vi "HydroHeader.vi"(0 "Comment":string, 1 "Scope":bool, 2 "File Name In":string, 3 "Votage scaling":T1={"Digitizer (dB)"=26.0, "Gain (dB)"=0.0, "Atten (dB)"=0.0}) -> (5 "Header String Out":string)   [LabVIEW 2022 SP3]
uses:
  ViewData/-ReadEye/Header.ctl
  ScanningControl/Digitizers/GaGe/-GageUtils/GageGlobals.vi
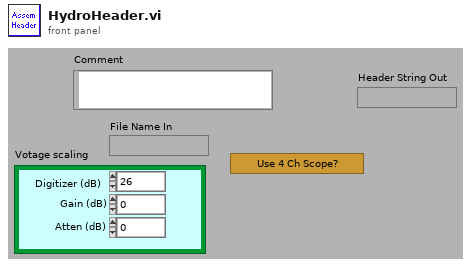
[diagram p1: front panel]
types:
  T1 = cluster{"Digitizer (dB)":sgl, "Gain (dB)":sgl, "Atten (dB)":sgl}
  T2 = typedef "Header.ctl" = cluster{"header info":cluster{"Header":string, "Head length":i16}, "A/D info":cluster{"# rf points per line":u16, "# lines per scan":u16, "sample rate MHz":u16, "# A/D bits":i16, "# bytes per A/D":u16, "TGC Flag":u16, "A/D Type":string}, "Tranducer Info":cluster{"bandwidth":sgl, "center freq":sgl, "start freq":sgl, "ID":i32}, "Scan Info":cluster{"delay":sgl, "pivot distance":sgl, "sector scan angle":sgl, "operator":string, "Scan Mode":string, "location":string}, "Time/Date Info":cluster{"date":string, "time":string}, "RF Info":cluster{"RF file name":string, "RF file att":string, "RF cal file name":string, "RF cal file att":string}, "Patient Info":cluster{"ID":string, "extended ID":string, "age":u16, "sex":string, "previously\nscanned":string, "PSA":sgl, "LOS":u8, "Ethnicty 2":u8, "Race":u8}, "Tissue Type":cluster{"organ":i16, "disease type":i16, "disease location":i16, "IQ_pts":u16, "RcvBuffer":u8, "RcvFrame":u16, "IQBuff":u8, "IQFrame":u16, "IQPage":u8}, "Votage scaling":cluster{"Digitizer (dB)":sgl, "Gain (dB)":sgl, "Atten (dB)":sgl}, "Comment":string, "Misc Info":cluster{"avg num":u16, "c speed":i16, "Div By or SF zones":i16, "XMIT CHS":u8, "RCV CHS":u8, "Xmit angle":sgl}, "Therapy Parameters":cluster{"Theraputic Freq (MHz)":sgl, "Time on (s)":sgl, "Therapy amplitude (mV)":sgl, "Lines Before":u16, "Lines After":u16}, "Scan Settings":cluster{"Energy (uJ or V)":u8, "Damp (Ohm) or Fc":u8, "HP Filt (KHz)":u8, "LP Filt (MHz)":u8, "Gain (db)":u8, "prf (kHz)":sgl, "Distance between\nscan lines (um)":u16, "Distance between\nscan planes (um)":u16, "Scan line gap (um)":sgl, "Scan plane gap (um)":sgl}, "Compression Parameters":cluster{"F1 (MHz)":sgl, "F2 (MHz)":sgl, "% taper":sgl, "duration":sgl}, "Patient Info Xtra":cluster{"First Name":string, "Last Name":string, "Notes":string}, "ROI Box":u16[]}
  T3 = cluster{"organ":i16, "disease type":i16, "disease location":i16}
  T4 = cluster{"bandwidth":sgl, "center freq":sgl, "start freq":sgl, "ID":i32}
  T5 = cluster{"# rf points per line":u16, "# lines per scan":u16, "sample rate MHz":u16, "# A/D bits":i16, "# bytes per A/D":u16, "TGC Flag":u16, "A/D Type":string}
  T6 = cluster{"Energy (microJ)":i32, "Energy (microJ)":i32, "Energy (microJ)":i32, "Energy (microJ)":i32, "Energy (microJ)":i32, "number":sgl, "number":i16, "number":i16}
  T7 = cluster{"F1 (MHz)":sgl, "F2 (MHz)":sgl, "Tukey taper":sgl, "duration":sgl}
  T8 = cluster{"delay":sgl, "pivot distance":sgl, "sector scan angle":sgl, "operator":string, "Scan Mode":string, "location":string}
  T9 = cluster{"ID":string, "extended ID":string, "age":u16, "sex":string, "previously\nscanned":string, "PSA":sgl, "LOS":u8, "Ethnicty 2":u8, "Race":u8}
  T10 = cluster{"RF file name":string, "RF file att":string, "RF cal file name":string, "RF cal file att":string}
  T11 = cluster{"avg num":i16, "c speed":i16, "Div By or SF zones":i16, "XMIT CHS":u8, "RCV CHS":u8}
  T12 = cluster{"Theraputic Freq (MHz)":sgl, "Time on (s)":sgl, "Therapy amplitude (mV)":sgl, "Lines Before":u16, "Lines After":u16}
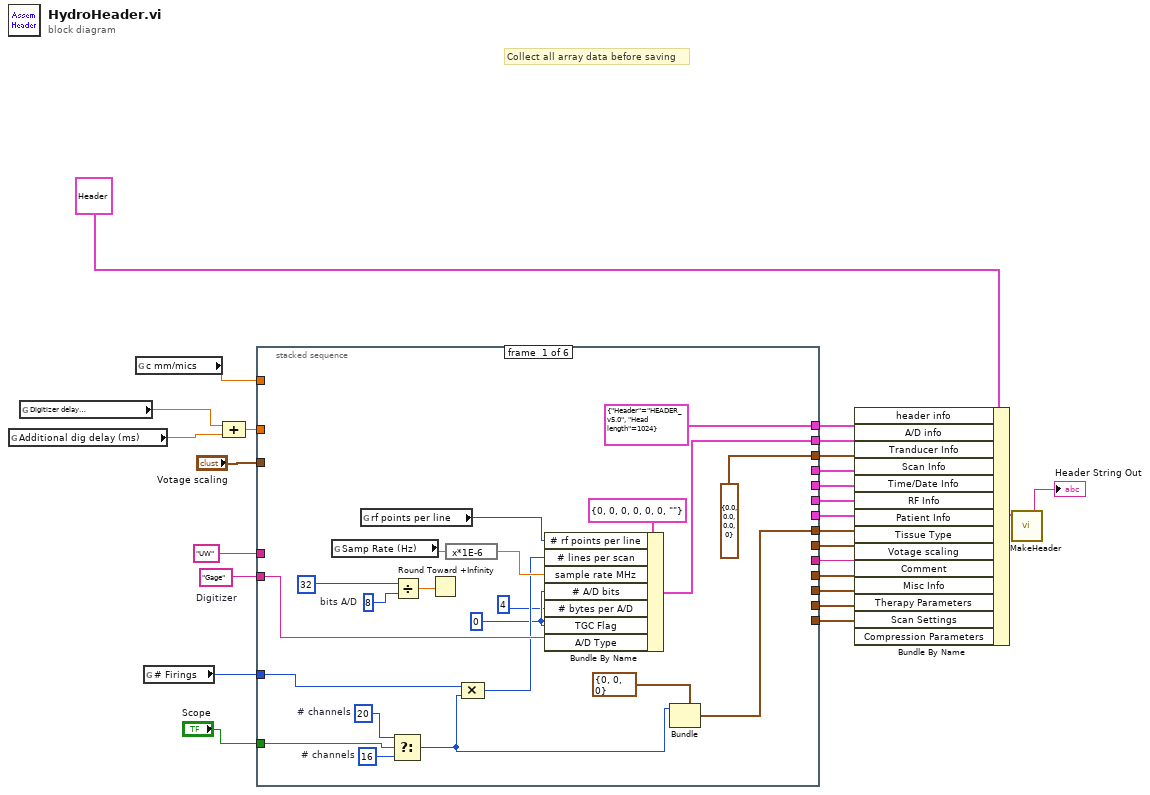
[diagram p0: block diagram]
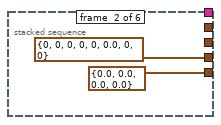
[diagram p2: hidden frame]
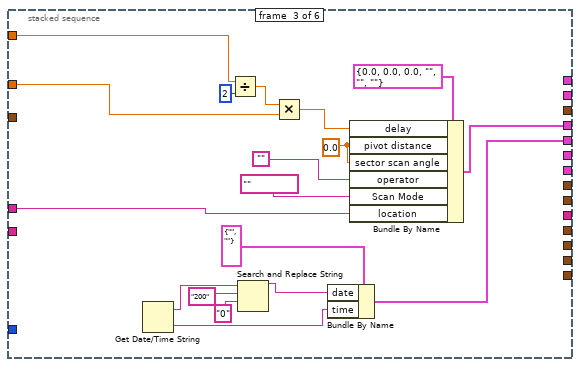
[diagram p3: hidden frame]
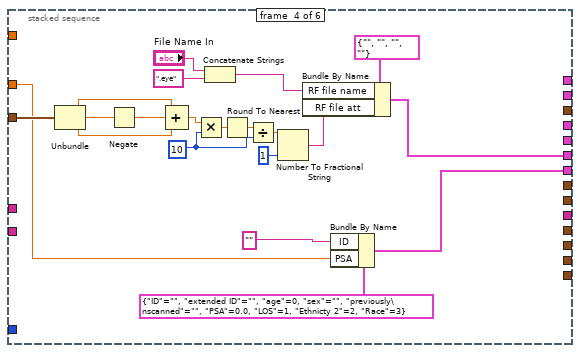
[diagram p4: hidden frame]
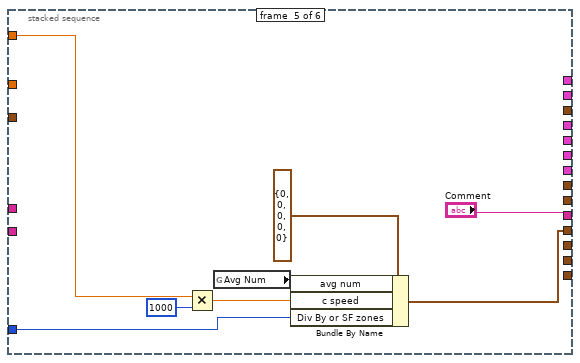
[diagram p5: hidden frame]
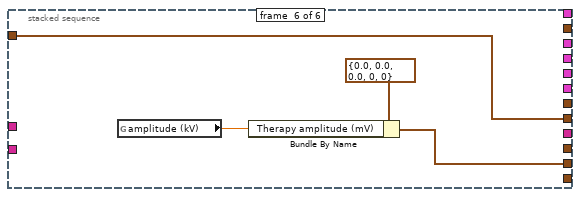
[diagram p6: hidden frame]
diagram:
  w21 = "Gage"  # Digitizer
  # "Collect all array data before saving"
  n1 = global read "GageGlobals.vi" "Additional dig delay (ms)"() -> (w4:dbl)
  n2 = global read "GageGlobals.vi" "Digitizer delay\n (ms)"() -> (w3:dbl)
  n3 = global read "GageGlobals.vi" "c mm/mics"() -> (w2:sgl)
  n4 = global read "GageGlobals.vi" "# Firings"() -> (w5:u16)
  n5 = Compound Arithmetic op=ADD(w3, w4) -> (w15:dbl)
  n6 = stacked-sequence {
    tunnel: [cluster{"Header":string, "Head length":i16} {"Header"="HEADER_v5.0", "Head length"=1024} ("header info") _ _ _ _ _] -> w26
    tunnel: [w43 _ _ _ _ _] -> w24
    tunnel: "UW" -> [_ _ w59 _ _ _]
    tunnel: [_ _ w61 _ _ _] -> w22
    tunnel: w21 -> [w42 _ _ _ _ _]
    tunnel: [T4 {"bandwidth"=0.0, "center freq"=0.0, "start freq"=0.0, "ID"=0} ("Tranducer Info") _ _ _ _ _] -> w20
    tunnel: w2 -> [_ _ w58 _ w93 _]
    tunnel: [_ _ w53 _ _ _] -> w19
    tunnel: "Votage scaling" -> [_ _ _ w70 _ w98]
    tunnel: [_ _ _ w74 _ _] -> w16
    tunnel: w15 -> [_ _ w51 w69 _ _]
    tunnel: [_ _ _ w72 _ _] -> w14
    tunnel: [_ _ _ _ _ w98] -> w13
    tunnel: [w29 _ _ _ _ _] -> w12
    tunnel: [_ _ _ _ "Comment" _] -> w11
    tunnel: [_ _ _ _ w91 _] -> w10
    tunnel: [_ _ _ _ _ w99] -> w9
    tunnel: [_ T6 {"Energy (microJ)"=0, "Energy (microJ)"=0, "Energy (microJ)"=0, "Energy (microJ)"=0, "Energy (microJ)"=0, "number"=0.0, "number"=0, "number"=0} ("output cluster") _ _ _ _] -> w8
    tunnel: [_ T7 {"F1 (MHz)"=0.0, "F2 (MHz)"=0.0, "Tukey taper"=0.0, "duration"=0.0} ("Compression Parameters") _ _ _ _] -> w7
    tunnel: w5 -> [w38 _ _ _ w90 _]
    tunnel: "Scope" -> [w32 _ _ _ _ _]
    frame #0 {
      w33 = 20  # # channels
      w34 = 16  # # channels
      w28 = u16 0 ("TGC Flag")
      w44 = 8  # bits A/D
      n7 = global read "GageGlobals.vi" "Samp Rate (Hz)"() -> (w35:dbl)
      n8 = global read "GageGlobals.vi" "rf points per line"() -> (w36:i32)
      n9 = Select(t=w33, s=w32, f=w34) -> (s? t:f=w30:i32)
      n10 = Divide(x=32, y=w44) -> (x/y=w45:dbl)
      n11 = Round Toward +Infinity(x=w45) -> ()  [unwired: 1 out]
      n12 = expression code="x*1E-6"(w35) -> (w40:dbl)
      n13 = Compound Arithmetic op=MULTIPLY(w38, w30) -> (w37:i32)
      n14 = Bundle By Name(cluster=T5 {"# rf points per line"=0, "# lines per scan"=0, "sample rate MHz"=0, "# A/D bits"=0, "# bytes per A/D"=0, "TGC Flag"=0, "A/D Type"=""} ("A/D info"), "# rf points per line"=w36, "# lines per scan"=w37, "sample rate MHz"=w40, "# A/D bits"=w28, "# bytes per A/D"=u16 4 ("TGC Flag"), "TGC Flag"=w28, "A/D Type"=w42) -> (w43:T5)
      n15 = Bundle(cluster=T3 {"organ"=0, "disease type"=0, "disease location"=0} ("Tissue Type"), "organ"=w30) -> (w29:T3)  [unwired: 2 out]
    }
    frame #1 {
    }
    frame #2 {
      w52 = sgl 0.0 ("sector scan angle")
      n16 = Get Date/Time String() -> (date string=w65:string, time string=w63:string)  [unwired: 3 out]
      n17 = Divide(x=w58, y=2) -> (x/y=w57:sgl)
      n18 = Search and Replace String(input string=w65, search string="200", replace string="0") -> (result string=w62:string)  [unwired: 1 in, 7 out]
      n19 = Multiply(x=w57, y=w51) -> (x*y=w56:dbl)
      n20 = Bundle By Name(cluster=cluster{"date":string, "time":string} {"date"="", "time"=""} ("Time/Date Info"), "date"=w62, "time"=w63) -> (w61:cluster{"date":string, "time":string})
      n21 = Bundle By Name(cluster=T8 {"delay"=0.0, "pivot distance"=0.0, "sector scan angle"=0.0, "operator"="", "Scan Mode"="", "location"=""} ("Scan Info"), "delay"=w56, "pivot distance"=w52, "sector scan angle"=w52, "operator"="", "Scan Mode"="", "location"=w59) -> (w53:T8)
    }
    frame #3 {
      w86 = 10
      n22 = Unbundle(w70) -> ("Digitizer (dB)"=w82:sgl, "Gain (dB)"=w81:sgl, "Atten (dB)"=w80:sgl)
      n23 = Negate(x=w81) -> (-x=w71:sgl)
      n24 = Compound Arithmetic op=ADD(w82, w71, w80) -> (w79:sgl)
      n25 = Multiply(x=w79, y=w86) -> (x*y=w84:sgl)
      n26 = Concatenate Strings("File Name In", ".eye") -> (w75:string)
      n27 = Round To Nearest(number=w84) -> (nearest integer value=w83:sgl)
      n28 = Divide(x=w83, y=w86) -> (x/y=w85:sgl)
      n29 = Number To Fractional String(number=w85, precision (6)=i16 1) -> (F-format string=w78:string)  [unwired: 2 out]
      n30 = Bundle By Name(cluster=T10 {"RF file name"="", "RF file att"="", "RF cal file name"="", "RF cal file att"=""} ("RF Info"), "RF file name"=w75, "RF file att"=w78) -> (w74:T10)
      n31 = Bundle By Name(cluster=T9 {"ID"="", "extended ID"="", "age"=0, "sex"="", "previously\nscanned"="", "PSA"=0.0, "LOS"=1, "Ethnicty 2"=2, "Race"=3} ("Patient Info"), "ID"="", "PSA"=w69) -> (w72:T9)
    }
    frame #4 {
      n32 = Multiply(x=w93, y=1000) -> (x*y=w92:sgl)
      n33 = global read "GageGlobals.vi" "Avg Num"() -> (w89:i32)
      n34 = Bundle By Name(cluster=T11 {"avg num"=0, "c speed"=0, "Div By or SF zones"=0, "XMIT CHS"=0, "RCV CHS"=0} ("input cluster"), "avg num"=w89, "c speed"=w92, "Div By or SF zones"=w90) -> (w91:T11)
    }
    frame #5 {
      n35 = global read "GageGlobals.vi" "amplitude (kV)"() -> (w97:dbl)
      n36 = Bundle By Name(cluster=T12 {"Theraputic Freq (MHz)"=0.0, "Time on (s)"=0.0, "Therapy amplitude (mV)"=0.0, "Lines Before"=0, "Lines After"=0} ("Therapy Parameters"), "Therapy amplitude (mV)"=w97) -> (w99:T12)
    }
  }
  n37 = Bundle By Name(cluster=T2 {"header info"={"Header"="", "Head length"=0}, "A/D info"={"# rf points per line"=0, "# lines per scan"=0, "sample rate MHz"=0, "# A/D bits"=0, "# bytes per A/D"=0, "TGC Flag"=0, "A/D Type"=""}, "Tranducer Info"={"bandwidth"=0.0, "center freq"=0.0, "start freq"=0.0, "ID"=0}, "Scan Info"={"delay"=0.0, "pivot distance"=0.0, "sector scan angle"=0.0, "operator"="", "Scan Mode"="", "location"=""}, "Time/Date Info"={"date"="", "time"=""}, "RF Info"={"RF file name"="", "RF file att"="", "RF cal file name"="", "RF cal file att"=""}, "Patient Info"={"ID"="", "extended ID"="", "age"=0, "sex"="", "previously\nscanned"="", "PSA"=0.0, "LOS"=1, "Ethnicty 2"=3, "Race"=3}, "Tissue Type"={"organ"=0, "disease type"=0, "disease location"=0, "IQ_pts"=0, "RcvBuffer"=0, "RcvFrame"=0, "IQBuff"=0, "IQFrame"=0, "IQPage"=0}, "Votage scaling"={"Digitizer (dB)"=0.0, "Gain (dB)"=0.0, "Atten (dB)"=0.0}, "Comment"="", "Misc Info"={"avg num"=0, "c speed"=0, "Div By or SF zones"=0, "XMIT CHS"=0, "RCV CHS"=0, "Xmit angle"=0.0}, "Therapy Parameters"={"Theraputic Freq (MHz)"=0.1, "Time on (s)"=1.0, "Therapy amplitude (mV)"=50.0, "Lines Before"=20, "Lines After"=80}, "Scan Settings"={"Energy (uJ or V)"=0, "Damp (Ohm) or Fc"=0, "HP Filt (KHz)"=0, "LP Filt (MHz)"=0, "Gain (db)"=0, "prf (kHz)"=0.0, "Distance between\nscan lines (um)"=0, "Distance between\nscan planes (um)"=0, "Scan line gap (um)"=0.0, "Scan plane gap (um)"=0.0}, "Compression Parameters"={"F1 (MHz)"=0.0, "F2 (MHz)"=0.0, "% taper"=0.0, "duration"=0.0}, "Patient Info Xtra"={"First Name"="", "Last Name"="", "Notes"=""}, "ROI Box"=[0, 0, 0, 0]} ("Header In"), "header info"=w26, "A/D info"=w24, "Tranducer Info"=w20, "Scan Info"=w19, "Time/Date Info"=w22, "RF Info"=w16, "Patient Info"=w14, "Tissue Type"=w12, "Votage scaling"=w13, "Comment"=w11, "Misc Info"=w10, "Therapy Parameters"=w9, "Scan Settings"=w8, "Compression Parameters"=w7) -> (w18:T2)
  n38 = call "MakeHeader.vi"("Header In"=w18) -> ("Header String"=→"Header String Out":string)  [unwired: 6 out]
